vi "Directory Content.vi"(7 "Directory (\"\\\")":string="\\", 8 "error in (no error)":errorcluster, 11 "VISA resource name":refnum<visa-resource-name>) -> (0 "error out":errorcluster, 1 "Size":string[](array[string]), 2 "Name":string[](array[string]), 3 "VISA resource name out":refnum<visa-resource-name>, 4 "Free Size":dbl format="%#_12f", 5 "Used Size":dbl format="%#_12f")   [LabVIEW 2018, in "Agilent ENA Series.lvlib"]
doc: "Reads data from a file on the built-in storage device of the E5070B/E5071B/E5071C.\n\nBy reading out data with this VI and writing it to a file on the external controller, file transfer from the E5070B/E5071B/E5071C to the external controller can be realized. On the other hand, by reading out data from the external controller and writing it to a file on the E5070B/E5071B/E5071C with this funcition, file transfer from the external controller to the E5070B/E5071B/E5071C can be realized.\n\nSpecify the file name with the extension. If you want to specify \na file on the floppy disk\ndrive, you need to add \"A:\" at the beginning of the file name. When you use directory names and file name, separate them with \"/\" (slash) or \"\\\" (backslash)."
uses:
  Agilent ENA Series.lvlib
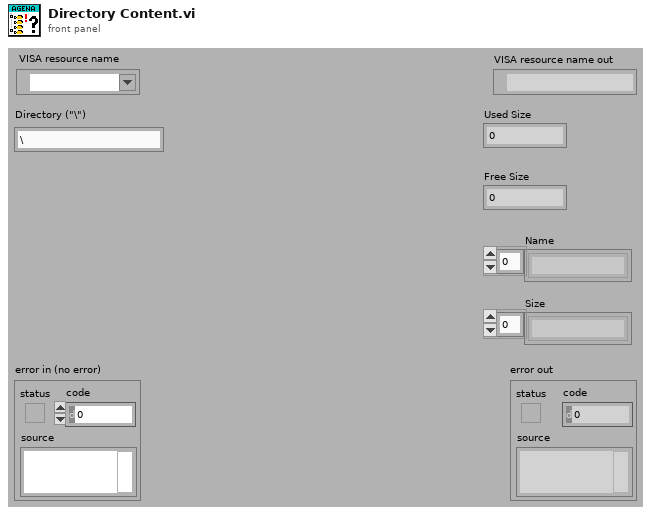
[diagram p1: front panel]
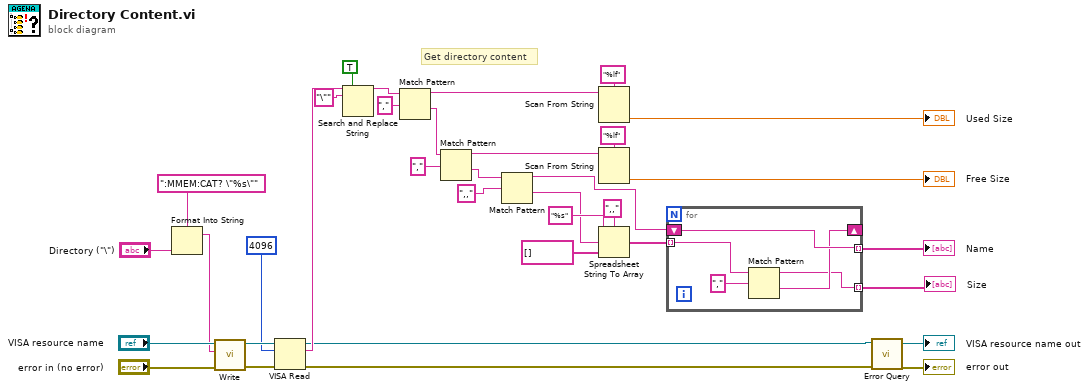
[diagram p0: block diagram]
diagram:
  # "Get directory content"
  n1 = Format Into String(format string=":MMEM:CAT? \"%s\"", "Directory (\"\\\")") -> (resulting string=w31:string)  [unwired: 2 in, 1 out]
  n2 = call "Write.vi"("error in (no error)"="error in (no error)", "String ()"=w31, "VISA resource name"="VISA resource name") -> ("error out"=w29:errorcluster, "VISA resource name out"=w30:refnum<visa-resource-name>)  [unwired: 6 in, 1 out]
  n3 = VISA Read(VISA resource name=w30, byte count=u32 4096, error in (no error)=w29) -> (VISA resource name out=w2:refnum<visa-resource-name>, read buffer=w15:string, error out=w1:errorcluster)  [unwired: 1 out]
  n4 = Search and Replace String(replace all?=TRUE ("replace all? (F)"), input string=w15, search string="\"") -> (result string=w12:string)  [unwired: 5 in, 3 out]
  n5 = Match Pattern(string=w12, regular expression=",") -> (before substring=w20:string, after substring=w22:string)  [unwired: 1 in, 2 out]
  n6 = Match Pattern(string=w22, regular expression=",") -> (before substring=w16:string, after substring=w9:string)  [unwired: 1 in, 2 out]
  n7 = Match Pattern(string=w9, regular expression=",," ("delimiter (Tab)")) -> (before substring=w5:string, after substring=w8:string)  [unwired: 1 in, 2 out]
  n8 = Scan From String(format string="%lf", input string=w20) -> (output 1=→"Used Size":dbl)  [unwired: 3 in, 3 out]
  n9 = Scan From String(format string="%lf", input string=w16) -> (output 1=→"Free Size":dbl)  [unwired: 3 in, 3 out]
  n10 = Spreadsheet String To Array(delimiter (Tab)=",,", format string="%s", spreadsheet string=w8, array type (2D Dbl)=string[] []) -> (array=w10:string[])
  n11 = for {
    tunnel: w10 -> [w40] mode=indexing
    shift-right: [w37] -> _
    shift-left: w5 -> [w38]
    tunnel: [w38] -> w7 mode=indexing
    tunnel: [w36] -> w6 mode=indexing
    n12 = Match Pattern(string=w40, regular expression="," ("delimiter (Tab)")) -> (before substring=w36:string, after substring=w37:string)  [unwired: 1 in, 2 out]
  }
  "Name" <- w7
  "Size" <- w6
  n13 = call "Error Query.vi"("error in (no error)"=w1, "VISA resource name"=w2) -> ("error out"=→"error out":errorcluster, "VISA resource name out"=→"VISA resource name out":refnum<visa-resource-name>)  [unwired: 6 in, 2 out]
